vi "AlliGator Draw Phasor Ratio References on Phasor Plot.vi"(8 "error in (no error)":errorcluster, 11 "Phasor Plot Refnum in":T1) -> (0 "error out":errorcluster, 3 "Phasor Plot Refnum out":T1)   [LabVIEW 2021, in "AlliGator Phasor Plot.lvlib"]
doc: "Does the actual drawing of Phasor Ratio References (and associated segment and boundary region) on the Phasor Plot image."
uses:
  AlliGator Phasor Plot.lvlib
  <vilib>/vision/Image Controls.llb/IMAQ Image.ctl
  AlliGator Variables List.ctl
  AlliGator Phasor Plot Reference Points.ctl
  AlliGator Settings List.ctl
  08c29e31-a428-4f06-8fa9-37cc1cf687de.vi
  a2f43300-ec38-48b4-b16a-acb1cf69b6dd.vi
  Variant/Variant to Data/Variant to DBL.vi
  Variant/Variant to Data/Variant to I32.vi
  Variant/Variant to Data/Variant to Boolean.vi
  AlliGator Globals, Variables & Constants.lvlib
  AlliGator Phasor Ratio.lvlib
  AlliGator Settings.lvlib
  Variant/Variant to Data/Variant to Data.lvlib
  Time/Time.lvlib
  Image/Image.lvlib
  Error/Error.lvlib
panel:
  out "elapsed (relative) seconds":dbl
  # "see the AlliGator License on the block diagram (Ctrl+E or Window:Show Block Diagram)"
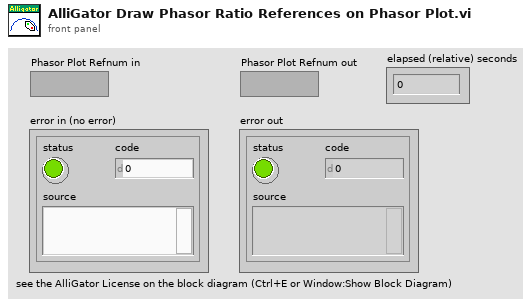
[diagram p1: front panel]
types:
  T1 = typedef "IMAQ Image.ctl" = refnum<image>
  T2 = typedef "AlliGator Settings.lvlib/AlliGator Settings List.ctl" = enum16{"GUI:Visible Settings Tab", "GUI:Last Run Version", "Source Image:Use Image Histogram for Contrast", "Source Image:Low Count Pixels Rejection Options", "Source Image:High Count Pixels Rejection Options", "Source Image:Use Image Brightness", "Source Image:Blend Overlay with Image Background", "Source Image:Use Fixed ROI Diameter", "Source Image:ROI Diameter", "Source Image:ROI Center Color", "Source Image:Peak Threshold", "Source Image:Intensity Threshold", "Source Image:Image Binning Options", "Source Image:Image Smoothing Options", "Source Image:Image Histogram Active", "Source Image:Invert Binary Mask", "Source Image:Hot Pixel Removal", "Source Image:Overlay Analyzed ROI Center", "Source Image:Auto-Adjust Contrast", "Source Image:Histogram Lower Percentile", "Source Image:Histogram Upper Percentile", "Source Image:Save Source Image", "Source Image:Scale Bar Options", "Source Image:Image Resolution (Pixel Size)", "Source Image:Flatfield Correction", "Source Image:Show Dead Left Columns Correction", "Source Image:Dead Left Columns Correction", "Source Image:Image Pre-Processing Operations Order", "Source Image:Overlay ROI Median", "Source Image:Median Overlay Color", "Data Information:Gate Width", "Data Information:Nanotime Gate Separation", "Data Information:Macrotime Gate Separation", "Data Information:Gate Step", "Data Information:# Gates", "Data Information:Gate Image Exposure", "Data Information:Gate Image Integration", "Data Information:Gates to Skip", "Data Information:Gates to Keep", "Data Information:Define Gates to", "Data Information:Channel Name", "Data Information:Available Channel Names", "Data Information:Channel Arithmetic", "Data Information:Background File Subtraction", "Data Information:Background File", "Data Information:Background Scaling Factor", "Data Information:Background Pile-up Correction", "Data Information:Background Pixel Well Capacity", "Data Information:Laser Period", "Data Information:SYNC Period", "Data Information:Pile-up Correction", "Data Information:Pixel Well Capacity", "Data Information:Dataset Scaling Factor", "Fluorescence Decay_Decay Pre-Processing:Reverse Gates", "Fluorescence Decay_Decay Pre-Processing:Verbose Decay Pre-Processing", "Fluorescence Decay_Decay Pre-Processing:Use Decay Pre-Processing", "Fluorescence Decay_Decay Pre-Processing:Background Subtraction", "Fluorescence Decay_Decay Pre-Processing:Background Definition Range", "Fluorescence Decay_Decay Pre-Processing:Baseline Subtraction Method", "Fluorescence Decay_Decay Pre-Processing:Decay Pre-Processing Operations Order", "Fluorescence Decay_Decay Pre-Processing:Smoothing Parameter", "Fluorescence Decay_Decay Pre-Processing:Shift Decay", "Fluorescence Decay_Decay Pre-Processing:Decay Shift Parameters", "Fluorescence Decay_Decay Pre-Processing:Fold Decay", "Fluorescence Decay_Decay Pre-Processing:# Folds", "Fluorescence Decay_Decay Pre-Processing:1-Normalize Decay", "Fluorescence Decay_Decay Pre-Processing:[0-1]-Normalize Decay", "Fluorescence Decay_Decay Pre-Processing:Smoothen Decay", "Fluorescence Decay_Decay Pre-Processing:Extrapolate Decay", "Fluorescence Decay_Decay Pre-Processing:Use Periodicity", "Fluorescence Decay_Decay Pre-Processing:Use Cursors", "Fluorescence Decay_Decay Pre-Processing:Tail Fraction", "Fluorescence Decay_Decay Pre-Processing:Head Fraction", "Fluorescence Decay_Decay Pre-Processing:Additional Points", "Fluorescence Decay_Decay Pre-Processing:Straighten Decay", "Fluorescence Decay_Decay Pre-Processing:Constant Background", "Fluorescence Decay_Decay Pre-Processing:Pixel-Normalize Decay", "Fluorescence Decay_Advanced Analysis:Extract IRF instead of Decay", "Fluorescence Decay_Advanced Analysis:IRF Extraction Options", "Fluorescence Decay_Advanced Analysis:IRF Optimization Options", "Fluorescence Decay_Advanced Analysis:Square Pulse Options", "Fluorescence Decay_Advanced Analysis:IRF Order", "Fluorescence Decay_Advanced Analysis:IRF Time Constants", "Fluorescence Decay_Advanced Analysis:Wavelet Analysis Options", "Fluorescence Decay_Advanced Analysis:Average Lifetime Options", "Fluorescence Decay_Fit Options:Fit Options", "Fluorescence Decay_Fit Options:Use Legacy Fitting Approach", "Fluorescence Decay_Fit Options:Use Data Information Laser Period", "Fluorescence Decay_Fit Parameters:Displayed Fit Parameters", "Fluorescence Decay_Fit Parameters:Fit Parameter Constraints", "Fluorescence Decay_Fit Parameters:Export Tabulated Results", "Fluorescence Decay_Fit Parameters:MLE Baseline Offset Type", "Fluorescence Decay_Fit Parameters:MLE Baseline Offset", "Fluorescence Decay_Fit Parameters:Guess Parameter Names", "Fluorescence Decay_Fit Parameters:Guess Parameter Values", "Fluorescence Decay_Fit Parameters:Guess Parameters Options", "Fluorescence Decay_Styles:Show Last Decay Only", "Fluorescence Decay_Styles:Decay Graph Color Array", "Fluorescence Decay:Decay Graph Active", "Fluorescence Decay Statistics:Min Peak Value", "Fluorescence Decay Statistics:Reject Low Decay Peak Pixels", "Fluorescence Decay Statistics:Reject High Decay Peak Pixels", "Fluorescence Decay Statistics:Max Peak Value", "Time Traces:Use File Timestamp", "Time Traces:Time Step", "Time Traces:Use Intensity Correction File", "Time Traces:Intensity Correction File", "Phasor Plot:Phasor Plot Smoothing Options", "Phasor Plot:Phasor Plot Size", "Phasor Plot:Phasor Plot Graphics Options", "Phasor Plot:Cumulative Phasor Plot", "Phasor Plot:Use Phasor Brightness", "Phasor Plot:Blend Overlay with Phasor Background", "Phasor Plot:Save Phasor Plot", "Phasor Plot:Show References", "Phasor Plot:Phasor Ratio Decay Range", "Phasor Plot:Exponential Fading", "Phasor Plot:Phasor Ratio Reference Colors", "Phasor Plot:Reference Radius", "Phasor Plot:Show Color Map Vertices", "Phasor Plot:Phasor Plot Active", "Phasor Plot:Phasor Ratio Color Map Type", "Phasor Plot:Phasor Ratio Color Map", "Phasor Plot:Phasor Ratio Display Range", "Phasor Plot:Selected Image ROI(s)", "Phasor Plot:All Image ROIs", "Phasor Plot:Selected Phasor Plot ROI(s)", "Phasor Plot:All Phasor Plot ROIs", "Phasor Plot:Phasor Ratio Color-Coded Quantity", "Phasor Plot:Store Phasor Harmonics", "Phasor Plot:Draw Reference Segment", "Phasor Plot:User-Defined Quantity", "Phasor Graph:Phasor Frequency", "Phasor Graph:Phasor Ratio Type", "Phasor Graph:Pixel-level Phasor Computation", "Phasor Graph:Save Phasor Graph", "Phasor Graph:Phasor Graph Active", "Phasor Graph:Phasor SDV Options", "Phasor Calibration:Use Backup Calibration if needed", "Phasor Graph:Define Shortest Lifetime as", "Phasor Calibration:Backup Calibration Type", "Phasor Calibration:Calibration Type", "Phasor Calibration:Calibration Lifetime", "Phasor Calibration:Calibration Map Algorithm", "Single-Exponential Phasor Locus (SEPL):Gate Parameters", "Single-Exponential Phasor Locus (SEPL):User-defined Gate", "Single-Exponential Phasor Locus (SEPL):User-defined IRF", "Single-Exponential Phasor Locus (SEPL):Phasor Parameters", "Single-Exponential Phasor Locus (SEPL):Decay & IRF Parameters", "Single-Exponential Phasor Locus (SEPL):Display Parameters", "Lifetime Analysis:Decay Analysis Parameters", "Lifetime Analysis:Lifetime Map Active", "Plugins:Python Settings", "Miscellaneous:Verbose Mode", "Miscellaneous:Beep after Script", "Miscellaneous:Saved Image File Format", "Miscellaneous:Exported Gate Image Settings", "Miscellaneous:Include Loading in Timing", "Miscellaneous:Verbose Settings Mode", "Miscellaneous:Histogram Options", "Miscellaneous:Beep on Error", "Miscellaneous:# Logical Processors Used", "Miscellaneous:ROI Description Max Characters", "Miscellaneous:Verbose Error Mode", "Miscellaneous:Transparent Mask Color"}
  T3 = cluster{"Reference 1":u32, "Reference 2":u32, "Boundary":u32}
  T4 = typedef "AlliGator Phasor Ratio.lvlib/AlliGator Phasor Plot Reference Points.ctl" = cluster{"O_h":dbl, "O_v":dbl, "1_h":dbl, "1_v":dbl}
  T5 = typedef "AlliGator Globals, Variables & Constants.lvlib/AlliGator Variables List.ctl" = enum16{"---- GUI ----", "GUI:Initialization Status", "GUI:State Indicators Refnum", "GUI:Original AlliGator Menu Items", "GUI:Current Action Loop State", "GUI:Script in progress", "GUI:Playback", "GUI:Loop Playback", "GUI:Search ROI Used", "GUI:Search ROI", "Decay Graph Max Legend Size", "Intensity Graph Max Legend Size", "Decay Statistics Graph Max Legend Size", "Phasor Graph Max Legend Size", "Phasor Ratio Graph Max Legend Size", "Lifetime Graph Max Legend Size", "---- Files ----", "Files:Export Dataset Frames as Individual Files", "Files:Show Batch Export Help Balloons", "Files:Frames in Dataset", "Files:ptu File Frame Start Indices", "Files:Current Frame in Dataset", "Files:Current Frame Timestamp", "Files:Dataset Loaded", "Files:Dataset Metadata", "Files:Dataset Channel", "Files:Dataset Data Description", "Files:Background Dataset Metadata", "Files:Background Dataset Channel", "Files:Background Dataset Data Description", "Files:Background File Subtraction", "Files:Background File Path", "Files:Background File Pile-up Correction", "Files:Background File Pixel Well Capacity", "Files:Background File Scaling Factor", "Files:Current Dataset Load Settings", "Files:Dataset Path", "Files:ICCD-specific Information", "Files:Macrotime Gate Separation", "------ Python Plugins ------", "Python Plugins:Information", "Python Plugins:Python Session", "Python Plugins:Valid Python Session?", "---- Source Image ----", "Source Image:ROIs", "Source Image:Current ROI", "Source Image:ROI Event Refnum", "X_Source Image Display Range", "X_Source Image Palette Information", "X_Type of Displayed Image", "X_Time Gate Slider", "Source Image:Palette List", "Source Image:Scale", "Source Image:ROI Overlay Color", "Source Image:Overlay to Erase", "Source Image:Is Displayed Image Accumulated", "Source Image:White Light Image Modified", "Source Image:Mask Image Modified", "---- Image Profile Window ----", "Image Profile:Window Event Refnum", "Image Profile:IntensityType", "Image Profile:Intensity Average Type", "Image Profile:Intensity-weighted SDV", "Image Profile:Box Profile Type", "Image Profile:Window Open", "Image Profile:Plotted Fit Parameter", "------ Phasor Graph -------", "Phasor Graph:Show Line", "---- Phasor Plot ---", "Phasor Plot:Parameters Changed", "Phasor Plot:FLI Dataset Modified since last Calculation", "Phasor Harmonics Data", "Selected Phasor Harmonics", "Phasor Harmonic Manager Event Refnum", "Phasor Plot:ROIs", "Phasor Plot:Current ROI", "Phasor Plot:ROI Event Refnum", "Phasor Plot:Image Reference Points", "Phasor Plot:Computed", "Phasor Plot:Palette Information", "Phasor Plot:Palette List", "Phasor Plot:Phasor Ratio Palette Information", "Phasor Plot:Phasor Ratio Palette List", "Phasor Plot:Image Scale", "Phasor Plot:Image Overlay to Erase", "Phasor Plot:Image Elements to Update", "Phasor Plot:Current Calculation Parameters", "Phasor Plot:Current Calibration Options", "Phasor Plot:Reset Cumulated Phasor Plot", "Phasor Plot:Reference 1", "Phasor Plot:Lifetime Reference 1", "Phasor Plot:Reference 1 Frequency", "Phasor Plot:Reference 2", "Phasor Plot:Lifetime Reference 2", "Phasor Plot:Reference 2 Frequency", "---- Decay Analysis ----", "Number of Selected Decays to Fit", "LS Fit Results", "LAR Fit Results", "BS Fit Results", "Last Decay Max - Min", "Best Fit Parameters", "Best Fit Parameter Names", "Actual Size X", "Actual Size Y", "Binning X", "Binning Y", "Actual # Gates", "Dataset Number", "Gates to...", "Gates Skipped", "Gates to keep", "Gate Step", "Gate Separation", "Reversed Gates", "Pile-up Correction", "Pixel Well Capacity", "Background Subtracted", "Background Subtraction Method", "Background Definition Range", "Background File (deprecated)", "Number of Dataset Accumulated", "Array of Accumulated Dataset Paths", "Do Averaged Datasets", "Destination File Path", "Process Plot Target", "Use 1/D as Phasor Frequency", "---- Decay Fit Parameter Map -----", "Decay Fit Parameter Map:Palette Information", "Decay Fit Parameter Map:Palette List", "------- Local Decay Window ---------", "Local Decay Graph Window:Event Refnum", "Local Decay Graph Window:Use normalized IRF for convolution", "----- Miscellaneous ----", "Misc:Skippable Dialog Windows Status"}
  T6 = typedef "Phasor.lvlib/Phasor (g, s).ctl" = cluster{"g":dbl, "s":dbl}
  T7 = cluster{"Left":i32, "Top":i32, "Right":i32, "Bottom":i32}
  T8 = cluster{"Phasor Plot x":dbl, "Phasor Plot y":dbl}
  T9 = cluster{"Phasor Plot x":dbl, "Phasor Plot y":dbl}[]
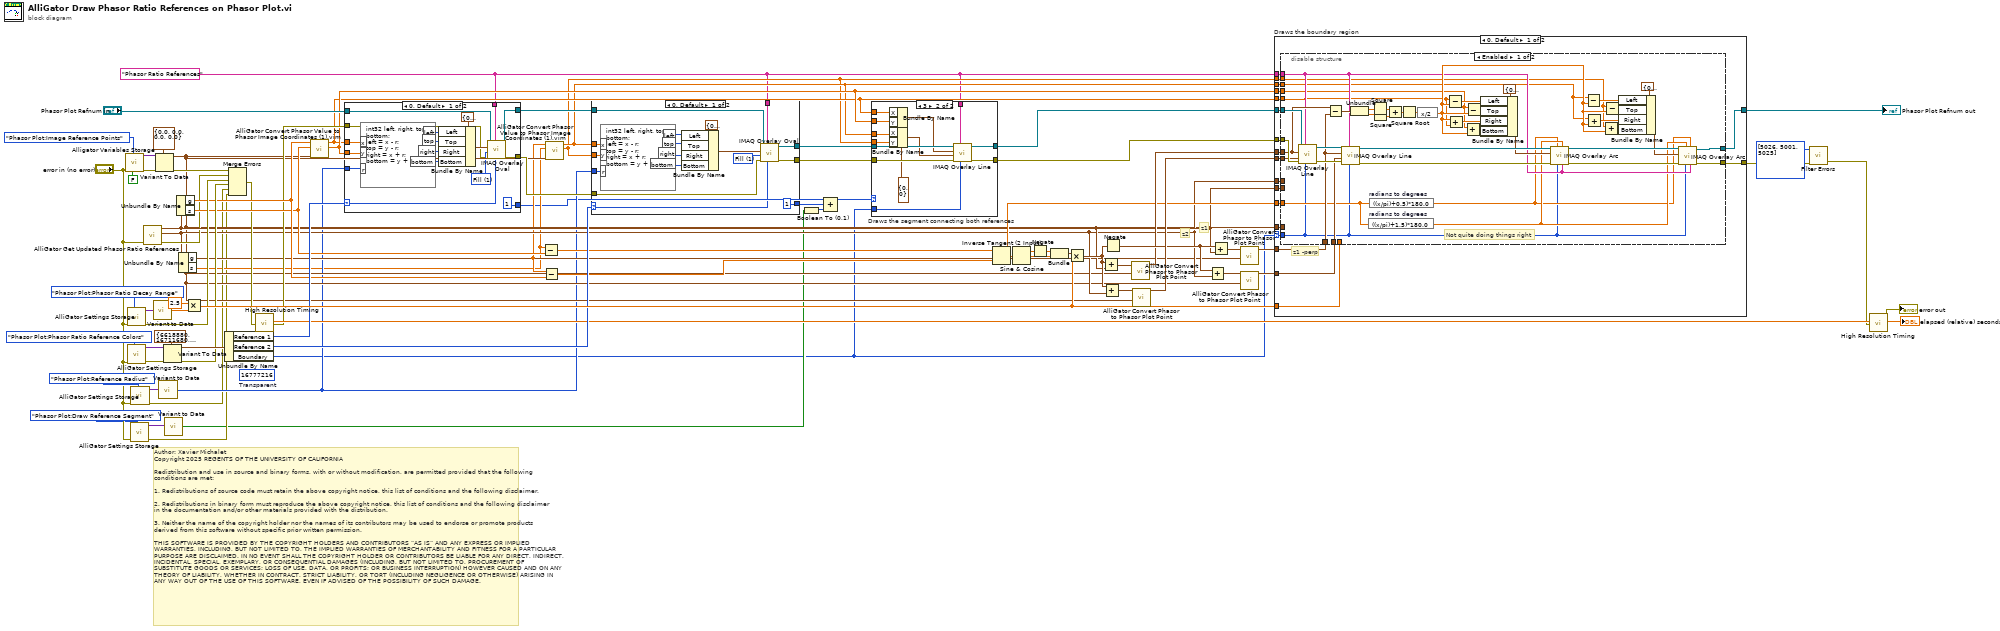
[diagram p0: block diagram]
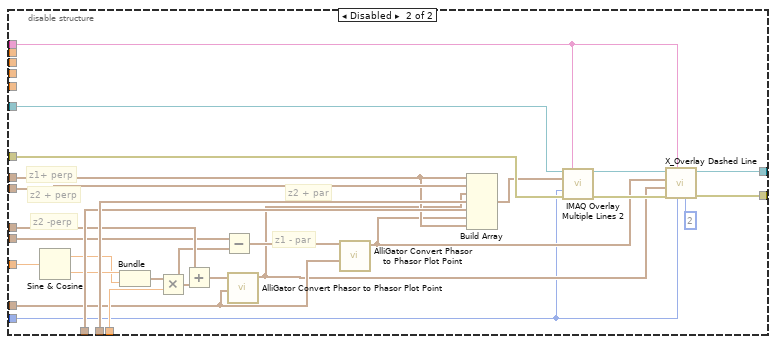
[diagram p3: hidden frame]
diagram:
  (unwired) u32 16777216  # Transparent
  w1 = "Phasor Ratio References" ("Group")
  # "Author: Xavier Michalet\nCopyright 2025 REGENTS OF THE UNIVERSITY OF CALIFORNIA\n\nRedistribution and use in source and binary forms, with or without modification, are permitted provided that the following conditions are met:\n\n1. Redistributions of source code must retain the above copyright notice, this list of conditions and the following disclaimer.\n\n2. Redistributions in binary form must reproduce the above copyright notice, this list of conditions and the following disclaimer in the documentation and/or other materials provided with the distribution.\n\n3. Neither the name of the copyright holder nor the names of its contributors may be used to endorse or promote products derived from this software without specific prior written permission.\n\nTHIS SOFTWARE IS PROVIDED BY THE COPYRIGHT HOLDERS AND CONTRIBUTORS “AS IS” AND ANY EXPRESS OR IMPLIED WARRANTIES, INCLUDING, BUT NOT LIMITED TO, THE IMPLIED WARRANTIES OF MERCHANTABILITY AND FITNESS FOR A PARTICULAR PURPOSE ARE DISCLAIMED. IN NO EVENT SHALL THE COPYRIGHT HOLDER OR CONTRIBUTORS BE LIABLE FOR ANY DIRECT, INDIRECT, INCIDENTAL, SPECIAL, EXEMPLARY, OR CONSEQUENTIAL DAMAGES (INCLUDING, BUT NOT LIMITED TO, PROCUREMENT OF SUBSTITUTE GOODS OR SERVICES; LOSS OF USE, DATA, OR PROFITS; OR BUSINESS INTERRUPTION) HOWEVER CAUSED AND ON ANY THEORY OF LIABILITY, WHETHER IN CONTRACT, STRICT LIABILITY, OR TORT (INCLUDING NEGLIGENCE OR OTHERWISE) ARISING IN ANY WAY OUT OF THE USE OF THIS SOFTWARE, EVEN IF ADVISED OF THE POSSIBILITY OF SUCH DAMAGE."
  # "z2"
  # "z1"
  n1 = call "Alligator Variables Storage.vi"("Get(F)/Set"=FALSE, "AlliGator Variable"=AlliGator_Variables_List."Phasor Plot:Image Reference Points" ("Alligator Variable"), "Error In"="error in (no error)") -> ("Error Out"=w78:errorcluster, "Data out"=w79:variant)  [unwired: 6 in, 1 out]
  n2 = call "AlliGator Settings Storage.vi"("AlliGator Settings List"=AlliGator_Settings_List."Phasor Plot:Phasor Ratio Decay Range", "Error In"="error in (no error)") -> ("Error Out"=w58:errorcluster, "Variant Data out"=w74:variant)  [unwired: 8 in]
  n3 = call "AlliGator Settings Storage.vi"("AlliGator Settings List"=AlliGator_Settings_List."Phasor Plot:Phasor Ratio Reference Colors", "Error In"="error in (no error)") -> ("Error Out"=w66:errorcluster, "Variant Data out"=w68:variant)  [unwired: 8 in]
  n4 = call "AlliGator Settings Storage.vi"("AlliGator Settings List"=AlliGator_Settings_List."Phasor Plot:Draw Reference Segment", "Error In"="error in (no error)") -> ("Error Out"=w16:errorcluster, "Variant Data out"=w18:variant)  [unwired: 8 in]
  n5 = call "AlliGator Settings Storage.vi"("AlliGator Settings List"=AlliGator_Settings_List."Phasor Plot:Reference Radius", "Error In"="error in (no error)") -> ("Error Out"=w25:errorcluster, "Variant Data out"=w27:variant)  [unwired: 8 in]
  n6 = call "AlliGator Get Updated Phasor Ratio References.vi"("error in (no error)"="error in (no error)") -> ("error out"=w31:errorcluster, "Phasor Ratio Reference 2"=w30:T6, "Phasor Ratio Reference 1"=w32:T6)  [unwired: 8 in]
  n7 = call-poly "Variant to Data.vi"("Variant"=w74) -> ("Value"=w71:dbl)  [unwired: 8 in]
  n8 = Variant To Data(error in=w78, type=T4 {"O_h"=0.0, "O_v"=0.0, "1_h"=0.0, "1_v"=0.0} ("Phasor Plot Reference Points"), Variant=w79) -> (data=w29:T4, error out=w59:errorcluster)
  n9 = call-poly "Variant to Data.vi"("Variant"=w27) -> ("Value"=w26:i32)  [unwired: 8 in]
  n10 = Variant To Data(error in=w66, type=T3 {"Reference 1"=6618880, "Reference 2"=16711680, "Boundary"=16776960} ("Phasor Ratio Reference Colors"), Variant=w68) -> (data=w65:T3, error out=w57:errorcluster)
  n11 = call-poly "Variant to Data.vi"("Variant"=w18) -> ("Value"=w15:bool)  [unwired: 8 in]
  n12 = Unbundle By Name(w32) -> ("g"=w55:dbl, "s"=w54:dbl)
  n13 = Unbundle By Name(w30) -> ("g"=w21:dbl, "s"=w20:dbl)
  n14 = Multiply(x=2.5, y=w71) -> (x*y=w70:dbl)
  n15 = Unbundle By Name(w65) -> ("Reference 1"=w64:u32, "Reference 2"=w63:u32, "Boundary"=w10:u32)
  n16 = Merge Errors(w59, w31, w58, w57, w25, w16) -> (w36:errorcluster)
  n17 = call "High Resolution Timing.vi"("Error In"=w36) -> ("elapsed (relative) seconds"=w62:dbl, "Error Out"=w35:errorcluster)  [unwired: 16 in, 1 out]
  n18 = call "AlliGator Convert Phasor Value to Phasor Image Coordinates (1).vim"("Phasor Plot Reference Points"=w29, "Phasor s"=w54, "Phasor g"=w55) -> ("Phasor Plot y"=w9:dbl, "Phasor Plot x"=w4:dbl)  [unwired: 7 in]
  n19 = case shown="0, Default" w64 {
    selector: w64 -> [w97 _]
    tunnel: w1 -> [w96 _]
    tunnel: "Phasor Plot Refnum in" -> [w95 w99]
    tunnel: [w91 w99] -> w56
    tunnel: w35 -> [w90 w98]
    tunnel: [w89 w98] -> w33
    tunnel: w4 -> [w88 _]
    tunnel: w9 -> [w87 _]
    tunnel: w26 -> [w82 _]
    tunnel: [1 ("Bottom") _] -> w12
    frame 0, Default {
      w94 = u32 1 items=["Frame", "Fill"] ("Drawing Mode (Frame)")
      n20 = formula code="int32 left, right, top, bottom;\nleft = x - r;\ntop = y - r;\nright = x + r;\nbottom = y + r;"("x"=w88, "y"=w87, "r"=w82) -> ("left"=w86:i32, "top"=w85:i32, "right"=w84:i32, "bottom"=w83:i32)
      n21 = Bundle By Name(cluster=T7 {"Left"=0, "Top"=0, "Right"=0, "Bottom"=0} ("Bounding Rectangle"), "Left"=w86, "Top"=w85, "Right"=w84, "Bottom"=w83) -> (w92:T7)
      n22 = call "IMAQ Overlay Oval"("Color"=w97, "Group"=w96, "error in (no error)"=w90, "Drawing Mode (Frame)"=w94, "Bounding Rectangle"=w92, "Image"=w95) -> ("error out"=w89:errorcluster, "Image Out"=w91:T1)  [unwired: 4 in]
    }
    frame 16777216 {
      # "transparent"
    }
  }
  n23 = Subtract(x=w20, y=w54) -> (x-y=w53:dbl)
  n24 = Subtract(x=w21, y=w55) -> (x-y=w52:dbl)
  n25 = call "AlliGator Convert Phasor Value to Phasor Image Coordinates (1).vim"("Phasor Plot Reference Points"=w29, "Phasor s"=w20, "Phasor g"=w21) -> ("Phasor Plot y"=w2:dbl, "Phasor Plot x"=w3:dbl)  [unwired: 7 in]
  n26 = case shown="0, Default" w63 {
    selector: w63 -> [w116 _]
    tunnel: w1 -> [w115 _]
    tunnel: w56 -> [w111 w117]
    tunnel: [w110 w117] -> w8
    tunnel: [w109 w118] -> w6
    tunnel: w33 -> [w108 w118]
    tunnel: w3 -> [w107 _]
    tunnel: w2 -> [w106 _]
    tunnel: w26 -> [w105 _]
    tunnel: [1 ("Bottom") _] -> w14
    frame 0, Default {
      w112 = u32 1 items=["Frame", "Fill"] ("Drawing Mode (Frame)")
      n27 = formula code="int32 left, right, top, bottom;\nleft = x - r;\ntop = y - r;\nright = x + r;\nbottom = y + r;"("x"=w107, "y"=w106, "r"=w105) -> ("left"=w104:i32, "top"=w103:i32, "right"=w102:i32, "bottom"=w101:i32)
      n28 = Bundle By Name(cluster=T7 {"Left"=0, "Top"=0, "Right"=0, "Bottom"=0} ("Bounding Rectangle"), "Left"=w104, "Top"=w103, "Right"=w102, "Bottom"=w101) -> (w114:T7)
      n29 = call "IMAQ Overlay Oval"("Color"=w116, "Group"=w115, "error in (no error)"=w108, "Drawing Mode (Frame)"=w112, "Bounding Rectangle"=w114, "Image"=w111) -> ("error out"=w109:errorcluster, "Image Out"=w110:T1)  [unwired: 4 in]
    }
    frame 16777216 {
      # "transparent"
    }
  }
  n30 = Boolean To (0,1)(Boolean=w15) -> (0, 1=w13:i16)
  n31 = Compound Arithmetic op=ADD(w12, w14, w13) -> (w11:i32)
  n32 = case "Draws the segment connecting both references" shown="3" w11 {
    tunnel: w10 -> [_ w129]
    tunnel: w9 -> [_ w127]
    tunnel: w8 -> [w120 w133]
    tunnel: [w120 w132] -> w7
    tunnel: w6 -> [w119 w131]
    tunnel: [w119 w130] -> w5
    tunnel: w4 -> [_ w128]
    tunnel: w3 -> [_ w126]
    tunnel: w2 -> [_ w125]
    tunnel: w1 -> [_ w121]
    frame 0, Default {
    }
    frame 3 {
      w124 = cluster{"X":i32, "Y":i32} {"X"=0, "Y"=0} ("Start Point")
      n33 = Bundle By Name(cluster=w124, "X"=w128, "Y"=w127) -> (w123:cluster{"X":i32, "Y":i32})
      n34 = Bundle By Name(cluster=w124, "X"=w126, "Y"=w125) -> (w122:cluster{"X":i32, "Y":i32})
      n35 = call "IMAQ Overlay Line"("Color"=w129, "Group"=w121, "error in (no error)"=w131, "End Point"=w122, "Start Point"=w123, "Image"=w133) -> ("error out"=w130:errorcluster, "Image Out"=w132:T1)  [unwired: 4 in]
    }
  }
  n36 = Inverse Tangent (2 Input)(1:w52, 2:w53) -> (0:w37:dbl)
  n37 = Sine & Cosine(0:w37) -> (1:w51:dbl, 2:w50:dbl)
  n38 = Negate(x=w51) -> (-x=w49:dbl)
  n39 = Bundle(w49, w50) -> (w48:cluster{dbl, dbl})  [unwired: 1 in]
  n40 = Multiply(x=w48, y=w70) -> (x*y=w47:cluster{dbl, dbl})
  n41 = Add(x=w47, y=w32) -> (x+y=w46:T6)
  n42 = Add(x=w47, y=w30) -> (x+y=w45:T6)
  n43 = Negate(x=w47) -> (-x=w42:cluster{dbl, dbl})
  n44 = call "AlliGator Convert Phasor to Phasor Plot Point.vi"("Phasor Plot Reference Points"=w29, "Phasor"=w46) -> ("Phasor Plot Point"=w39:T8)  [unwired: 9 in]
  n45 = call "AlliGator Convert Phasor to Phasor Plot Point.vi"("Phasor Plot Reference Points"=w29, "Phasor"=w45) -> ("Phasor Plot Point"=w44:T8)  [unwired: 9 in]
  n46 = Add(x=w42, y=w30) -> (x+y=w41:T6)
  n47 = Add(x=w42, y=w32) -> (x+y=w43:T6)
  n48 = call "AlliGator Convert Phasor to Phasor Plot Point.vi"("Phasor Plot Reference Points"=w29, "Phasor"=w43) -> ("Phasor Plot Point"=w38:T8)  [unwired: 9 in]
  n49 = call "AlliGator Convert Phasor to Phasor Plot Point.vi"("Phasor Plot Reference Points"=w29, "Phasor"=w41) -> ("Phasor Plot Point"=w40:T8)  [unwired: 9 in]
  n50 = case "Draws the boundary region" shown="0, Default" w10 {
    selector: w10 -> [w150 _]
    tunnel: [w152 w224] -> w72
    tunnel: w70 -> [w151 _]
    tunnel: w1 -> [w149 _]
    tunnel: w7 -> [w148 w224]
    tunnel: w5 -> [w147 w223]
    tunnel: w44 -> [w146 _]
    tunnel: w40 -> [w145 _]
    tunnel: w39 -> [w144 _]
    tunnel: w38 -> [w143 _]
    tunnel: w37 -> [w142 _]
    tunnel: [w141 w223] -> w23
    tunnel: w32 -> [w140 _]
    tunnel: w30 -> [w139 _]
    tunnel: w29 -> [w138 _]
    tunnel: w4 -> [w137 _]
    tunnel: w9 -> [w136 _]
    tunnel: w3 -> [w135 _]
    tunnel: w2 -> [w134 _]
    frame 0, Default {
      # "z1 -perp"
      n51 = disable-structure shown="Enabled" {
        disable-tunnel: w148 -> [w195 w207]
        disable-tunnel: w147 -> [w194 w206]
        disable-tunnel: w146 -> [w191 w222]
        disable-tunnel: w145 -> [w190 w221]
        disable-tunnel: w144 -> [w185 w219]
        disable-tunnel: w143 -> [w184 w220]
        disable-tunnel: w137 -> [w153 _]
        disable-tunnel: w136 -> [w154 _]
        disable-tunnel: w142 -> [w172 w218]
        disable-tunnel: w135 -> [w155 _]
        disable-tunnel: w134 -> [w156 _]
        disable-tunnel: w149 -> [w162 w203]
        disable-tunnel: [w161 w201] -> w141
        disable-tunnel: [w160 w200] -> w152
        disable-tunnel: w150 -> [w157 w197]
        disable-tunnel: w140 -> [_ w211]
        disable-tunnel: w151 -> [_ w214]
        disable-tunnel: w139 -> [_ w213]
        disable-tunnel: w138 -> [_ w208]
        frame Enabled {
          # "Not quite doing things right"
          n52 = call "IMAQ Overlay Line"("Color"=w157, "Group"=w162, "error in (no error)"=w194, "End Point"=w191, "Start Point"=w185, "Image"=w195) -> ("error out"=w192:errorcluster, "Image Out"=w193:T1)  [unwired: 4 in]
          n53 = Subtract(x=w185, y=w184) -> (x-y=w183:T8)
          n54 = call "IMAQ Overlay Line"("Color"=w157, "Group"=w162, "error in (no error)"=w192, "End Point"=w190, "Start Point"=w184, "Image"=w193) -> ("error out"=w188:errorcluster, "Image Out"=w189:T1)  [unwired: 4 in]
          n55 = Unbundle(w183) -> ("Phasor Plot x"=w182:dbl, "Phasor Plot y"=w181:dbl)
          n56 = expression code="((x/pi)+1.5)*180.0" "radians to degrees"(w172) -> (w159:dbl)
          n57 = expression code="((x/pi)+0.5)*180.0" "radians to degrees"(w172) -> (w158:dbl)
          n58 = Square(x=w182) -> (x^2=w180:dbl)
          n59 = Square(x=w181) -> (x^2=w179:dbl)
          n60 = Add(x=w180, y=w179) -> (x+y=w178:dbl)
          n61 = Square Root(x=w178) -> (sqrt(x)=w174:dbl)
          n62 = expression code="x/2"(w174) -> (w167:dbl)
          n63 = Subtract(x=w153, y=w167) -> (x-y=w177:dbl)
          n64 = Add(x=w167, y=w153) -> (x+y=w176:dbl)
          n65 = Add(x=w154, y=w167) -> (x+y=w173:dbl)
          n66 = Subtract(x=w154, y=w167) -> (x-y=w175:dbl)
          n67 = Bundle By Name(cluster=T7 {"Left"=0, "Top"=0, "Right"=0, "Bottom"=0} ("Bounding Rectangle"), "Left"=w177, "Top"=w175, "Right"=w176, "Bottom"=w173) -> (w186:T7)
          n68 = call "IMAQ Overlay Arc"("Group"=w162, "End Angle (degrees)"=w159, "Color"=w157, "Start Angle (degrees)"=w158, "error in (no error)"=w188, "Bounding Rectangle"=w186, "Image"=w189) -> ("error out"=w163:errorcluster, "Image Out"=w165:T1)  [unwired: 3 in]
          n69 = Subtract(x=w155, y=w167) -> (x-y=w168:dbl)
          n70 = Add(x=w155, y=w167) -> (x+y=w169:dbl)
          n71 = Add(x=w156, y=w167) -> (x+y=w171:dbl)
          n72 = Subtract(x=w156, y=w167) -> (x-y=w170:dbl)
          n73 = Bundle By Name(cluster=T7 {"Left"=0, "Top"=0, "Right"=0, "Bottom"=0} ("Bounding Rectangle"), "Left"=w168, "Top"=w170, "Right"=w169, "Bottom"=w171) -> (w164:T7)
          n74 = call "IMAQ Overlay Arc"("Group"=w162, "End Angle (degrees)"=w158, "Color"=w157, "Start Angle (degrees)"=w159, "error in (no error)"=w163, "Bounding Rectangle"=w164, "Image"=w165) -> ("error out"=w161:errorcluster, "Image Out"=w160:T1)  [unwired: 3 in]
        }
        frame Disabled {
          # "z2 + par"
          # "z1 - par"
          # "z1+ perp"
          # "z2 + perp"
          # "z2 -perp"
          n75 = Sine & Cosine(0:w218) -> (1:w216:dbl, 2:w217:dbl)
          n76 = Bundle(w217, w216) -> (w215:cluster{dbl, dbl})  [unwired: 1 in]
          n77 = Multiply(x=w215, y=w214) -> (x*y=w210:cluster{dbl, dbl})
          n78 = Add(x=w213, y=w210) -> (x+y=w212:T6)
          n79 = Subtract(x=w211, y=w210) -> (x-y=w209:T6)
          n80 = call "AlliGator Convert Phasor to Phasor Plot Point.vi"("Phasor Plot Reference Points"=w208, "Phasor"=w212) -> ("Phasor Plot Point"=w198:T8)  [unwired: 9 in]
          n81 = call "AlliGator Convert Phasor to Phasor Plot Point.vi"("Phasor Plot Reference Points"=w208, "Phasor"=w209) -> ("Phasor Plot Point"=w199:T8)  [unwired: 9 in]
          n82 = Build Array(w219, w222, w198, w221, w220, w199, w219) -> (w205:T9)
          n83 = call "IMAQ Overlay Multiple Lines 2"("Image"=w207, "Group"=w203, "Line End Points"=w205, "Color"=w197, "error in (no error)"=w206) -> ("Image Out"=w204:T1, "error out"=w202:errorcluster)  [unwired: 9 in]
          n84 = call "X_Overlay Dashed Line.vi"("Dash Length (0)"=u32 2, "Color"=w197, "Overlay Group"=w203, "error in (no error)"=w202, "Point 2"=w198, "Point 1"=w199, "Refnum in"=w204) -> ("error out"=w201:errorcluster, "Refnum out"=w200:T1)  [unwired: 3 in]
        }
      }
    }
    frame 16777216 {
      # "transparent"
    }
  }
  "Phasor Plot Refnum out" <- w72
  n85 = call "Filter Errors.vi"("Filtered Errors"=i32[] [5026, 5001, 5025], "error in (no error)"=w23) -> ("error out"=w22:errorcluster)  [unwired: 7 in]
  n86 = call "High Resolution Timing.vi"("relative seconds (NaN)"=w62, "Error In"=w22) -> ("elapsed (relative) seconds"=→"elapsed (relative) seconds":dbl, "Error Out"=→"error out":errorcluster)  [unwired: 15 in, 1 out]
